vi "Cleaned RTK Multiple String Capture Software.vi"() -> ()   [LabVIEW 2011]
uses:
  COM Port Control.ctl
  binary clusters control.ctl
  <vilib>/Utility/sysdir.llb/System Directory Type.ctl
panel:
  out "shutdown blocker":bool
  in  "Tab Control":T1(tab)
  in  "Update setup":bool
  in  "shutdown":bool
  in  "Base File Path":path caption="Base File Path (Destination that all RCVR files will be saved in)"
  in  "Time between samples (seconds)":u32=5 min=1 max=600 step=1
  in  "Number of hours to collect before starting new file":u16=1 min=1 max=24 step=1
  in  "Grennich Offset":dbl=-8.0 caption="Greenwich offset (hours)" min=-12.0 max=12.0 step=1.0
  in  "UPDT COM 1":bool
  in  "Use RCVR 1":bool caption="Use RCVR"
  in  "Name of RCVR 1":string="RCVR 1" caption="Name of RCVR"
  in  "COM Port 1":T2={"flow control"=0, "COM Port"="", "parity"=enum."None", "data bits"=8, "baud rate"=9600} {"data bits" min=5 max=8 step=1; "flow control" items=["None", "XON/XOFF", "RTS/CTS", "XON/XOFF & RTS/CTS", "DTR/DSR", "XON/XOFF & DTR/DSR"]}
  out "Last 10 RCVR 1":string[](array[string])
  in  "A_Off R 1":dbl caption="Antenna offset (meters)" max=0.0 format="%.4g"
  in  "Name of RCVR 2":string="RCVR 2" caption="Name of RCVR"
  in  "UPDT COM 2":bool
  out "Last 10 RCVR 2":string[](array[string])
  in  "COM Port 2":T2={"flow control"=0, "COM Port"="", "parity"=enum."None", "data bits"=8, "baud rate"=9600} {"data bits" min=5 max=8 step=1; "flow control" items=["None", "XON/XOFF", "RTS/CTS", "XON/XOFF & RTS/CTS", "DTR/DSR", "XON/XOFF & DTR/DSR"]}
  in  "Use RCVR 2":bool caption="Use RCVR"
  in  "A_Off R 2":dbl caption="Antenna offset (meters)" max=0.0 format="%.4g"
  in  "Name of RCVR 3":string="RCVR 3" caption="Name of RCVR"
  in  "UPDT COM 3":bool
  out "Last 10 RCVR 3":string[](array[string])
  in  "COM Port 3":T2={"flow control"=0, "COM Port"="", "parity"=enum."None", "data bits"=8, "baud rate"=9600} {"data bits" min=5 max=8 step=1; "flow control" items=["None", "XON/XOFF", "RTS/CTS", "XON/XOFF & RTS/CTS", "DTR/DSR", "XON/XOFF & DTR/DSR"]}
  in  "Use RCVR 3":bool caption="Use RCVR"
  in  "A_Off R 3":dbl caption="Antenna offset (meters)" max=0.0 format="%.4g"
  in  "Name of RCVR 4":string="RCVR 4" caption="Name of RCVR"
  in  "UPDT COM 4":bool
  out "Last 10 RCVR 4":string[](array[string])
  in  "COM Port 4":T2={"flow control"=0, "COM Port"="", "parity"=enum."None", "data bits"=8, "baud rate"=9600} {"data bits" min=5 max=8 step=1; "flow control" items=["None", "XON/XOFF", "RTS/CTS", "XON/XOFF & RTS/CTS", "DTR/DSR", "XON/XOFF & DTR/DSR"]}
  in  "Use RCVR 4":bool caption="Use RCVR"
  in  "A_Off R 4":dbl caption="Antenna offset (meters)" max=0.0 format="%.4g"
  in  "Name of RCVR 5":string="RCVR 5" caption="Name of RCVR"
  in  "UPDT COM 5":bool
  out "Last 10 RCVR 5":string[](array[string])
  in  "COM Port 5":T2={"flow control"=0, "COM Port"="", "parity"=enum."None", "data bits"=8, "baud rate"=9600} {"data bits" min=5 max=8 step=1; "flow control" items=["None", "XON/XOFF", "RTS/CTS", "XON/XOFF & RTS/CTS", "DTR/DSR", "XON/XOFF & DTR/DSR"]}
  in  "A_Off R 5":dbl caption="Antenna offset (meters)" max=0.0 format="%.4g"
  in  "Use RCVR 5":bool caption="Use RCVR"
  in  "Name of RCVR 6":string="RCVR 6" caption="Name of RCVR"
  in  "UPDT COM 6":bool
  out "Last 10 RCVR 6":string[](array[string])
  in  "COM Port 6":T2={"flow control"=0, "COM Port"="", "parity"=enum."None", "data bits"=8, "baud rate"=9600} {"data bits" min=5 max=8 step=1; "flow control" items=["None", "XON/XOFF", "RTS/CTS", "XON/XOFF & RTS/CTS", "DTR/DSR", "XON/XOFF & DTR/DSR"]}
  in  "A_Off R 6":dbl caption="Antenna offset (meters)" max=0.0 format="%.4g"
  in  "Use RCVR 6":bool caption="Use RCVR"
  in  "Name of RCVR 7":string="RCVR 7" caption="Name of RCVR"
  in  "UPDT COM 7":bool
  out "Last 10 RCVR 7":string[](array[string])
  in  "COM Port 7":T2={"flow control"=0, "COM Port"="", "parity"=enum."None", "data bits"=8, "baud rate"=9600} {"data bits" min=5 max=8 step=1; "flow control" items=["None", "XON/XOFF", "RTS/CTS", "XON/XOFF & RTS/CTS", "DTR/DSR", "XON/XOFF & DTR/DSR"]}
  in  "A_Off R 7":dbl caption="Antenna offset (meters)" max=0.0 format="%.4g"
  in  "Use RCVR 7":bool caption="Use RCVR"
  in  "Name of RCVR 8":string="RCVR 8" caption="Name of RCVR"
  in  "UPDT COM 8":bool
  out "Last 10 RCVR 8":string[](array[string])
  in  "COM Port 8":T2={"flow control"=0, "COM Port"="", "parity"=enum."None", "data bits"=8, "baud rate"=9600} {"data bits" min=5 max=8 step=1; "flow control" items=["None", "XON/XOFF", "RTS/CTS", "XON/XOFF & RTS/CTS", "DTR/DSR", "XON/XOFF & DTR/DSR"]}
  in  "A_Off R 8":dbl caption="Antenna offset (meters)" max=0.0 format="%.4g"
  in  "Use RCVR 8":bool caption="Use RCVR"
  in  "Name of RCVR 9":string="RCVR 9" caption="Name of RCVR"
  in  "UPDT COM 9":bool
  out "Last 10 RCVR 9":string[](array[string])
  in  "COM Port 9":T2={"flow control"=0, "COM Port"="", "parity"=enum."None", "data bits"=8, "baud rate"=9600} {"data bits" min=5 max=8 step=1; "flow control" items=["None", "XON/XOFF", "RTS/CTS", "XON/XOFF & RTS/CTS", "DTR/DSR", "XON/XOFF & DTR/DSR"]}
  in  "A_Off R 9":dbl caption="Antenna offset (meters)" max=0.0 format="%.4g"
  in  "Use RCVR 9":bool caption="Use RCVR"
  in  "Name of RCVR 10":string="RCVR 10" caption="Name of RCVR"
  in  "UPDT COM 10":bool
  out "Last 10 RCVR 10":string[](array[string])
  in  "COM Port 10":T2={"flow control"=0, "COM Port"="", "parity"=enum."None", "data bits"=8, "baud rate"=9600} {"data bits" min=5 max=8 step=1; "flow control" items=["None", "XON/XOFF", "RTS/CTS", "XON/XOFF & RTS/CTS", "DTR/DSR", "XON/XOFF & DTR/DSR"]}
  in  "A_Off R 10":dbl caption="Antenna offset (meters)" max=0.0 format="%.4g"
  in  "Use RCVR 10":bool caption="Use RCVR"
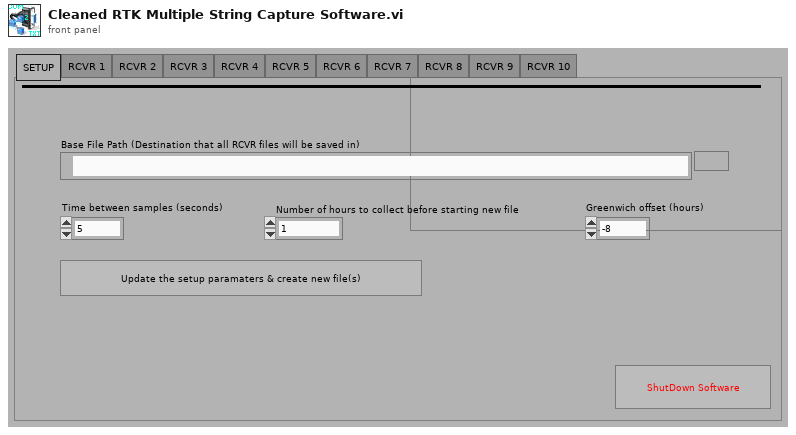
[diagram p1: front panel]
types:
  T1 = enum32{"SETUP", "RCVR 1", "RCVR 2", "RCVR 3", "RCVR 4", "RCVR 5", "RCVR 6", "RCVR 7", "RCVR 8", "RCVR 9", "RCVR 10"}
  T2 = typedef "COM Port Control.ctl" = cluster{"flow control":u16, "COM Port":refnum<visa-resource-name>, "parity":enum16{"None", "Odd", "Even", "Mark", "Space"}, "data bits":u16, "baud rate":u32}
  T3 = typedef "binary clusters control.ctl" = cluster{"setup save cluster":cluster{"Base File Path":path, "Time between samples (seconds)":u32, "Number of hours To Collect before starting new file ":u16, "Grennich Offset":dbl}, "RCVR1 Save Cluster":cluster{"Use RCVR 1":bool, "COM Port 1":T2, "Name of RCVR 1":string, "Antenna offset RCVR 1":dbl}, "RCVR2 Save cluster":cluster{"Use RCVR 2":bool, "COM Port 2":T2, "Name of RCVR 2":string, "Antenna offset RCVR 2":dbl}, "RCVR3 Save Cluster":cluster{"Use RCVR 3":bool, "Name of RCVR 3":string, "COM Port 3":T2, "Antenna offset RCVR 3":dbl}, "RCVR4 Save Cluster":cluster{"Use RCVR 4":bool, "Name of RCVR 4":string, "COM Port 4":T2, "Antenna offset RCVR 4":dbl}, "RCVR5 Save Cluster":cluster{"Use RCVR 5":bool, "Name of RCVR 5":string, "COM Port 5":T2, "Antenna offset RCVR 5":dbl}, "RCVR6 Save Cluster":cluster{"Use RCVR 6":bool, "Name of RCVR 6":string, "COM Port 6":T2, "Antenna offset RCVR 6":dbl}, "RCVR7 Save Cluster":cluster{"Use RCVR 7":bool, "Name of RCVR 7":string, "COM Port 7":T2, "Antenna offset RCVR 7":dbl}, "RCVR8 Save Cluster":cluster{"Use RCVR 8":bool, "Name of RCVR 8":string, "COM Port 8":T2, "Antenna offset RCVR 8":dbl}, "RCVR9 Save Cluster":cluster{"Use RCVR 9":bool, "Name of RCVR 9":string, "COM Port 9":T2, "Antenna offset RCVR 9":dbl}, "RCVR10 Save Cluster":cluster{"Use RCVR 10":bool, "Name of RCVR 10":string, "COM Port 10":T2, "Antenna offset RCVR 10":dbl}}
  T4 = enum16{"big-endian, network order", "native, host order", "little-endian"}
  T5 = cluster{"Number of hours To Collect before starting new file ":u16, "Base File Path":path, "Update setup":bool, "Shutdown software":bool, "Time between samples (seconds)":u32}
  T6 = typedef "System Directory Type.ctl" = i32
  T7 = cluster{"Base File Path":path, "Time between samples (seconds)":u32, "Number of hours To Collect before starting new file ":u16, "Grennich Offset":dbl}
  T8 = cluster{"Use RCVR 10":bool, "Name of RCVR 10":string, "COM Port 10":T2, "Antenna offset RCVR 10":dbl}
  T9 = cluster{"Use RCVR 1":bool, "COM Port 1":T2, "Name of RCVR 1":string, "Antenna offset RCVR 1":dbl}
  T10 = cluster{"Use RCVR 3":bool, "Name of RCVR 3":string, "COM Port 3":T2, "Antenna offset RCVR 3":dbl}
  T11 = cluster{"Use RCVR 4":bool, "Name of RCVR 4":string, "COM Port 4":T2, "Antenna offset RCVR 4":dbl}
  T12 = cluster{"Use RCVR 5":bool, "Name of RCVR 5":string, "COM Port 5":T2, "Antenna offset RCVR 5":dbl}
  T13 = cluster{"Use RCVR 6":bool, "Name of RCVR 6":string, "COM Port 6":T2, "Antenna offset RCVR 6":dbl}
  T14 = cluster{"Use RCVR 7":bool, "Name of RCVR 7":string, "COM Port 7":T2, "Antenna offset RCVR 7":dbl}
  T15 = cluster{"Use RCVR 8":bool, "Name of RCVR 8":string, "COM Port 8":T2, "Antenna offset RCVR 8":dbl}
  T16 = cluster{"Use RCVR 9":bool, "Name of RCVR 9":string, "COM Port 9":T2, "Antenna offset RCVR 9":dbl}
  T17 = cluster{"Use RCVR 2":bool, "COM Port 2":T2, "Name of RCVR 2":string, "Antenna offset RCVR 2":dbl}
  T18 = enum32{"invalid app kind", "Development System", "Run Time System", "Student Edition", "Embedded LabVIEW", "Evaluation", "Custom"}
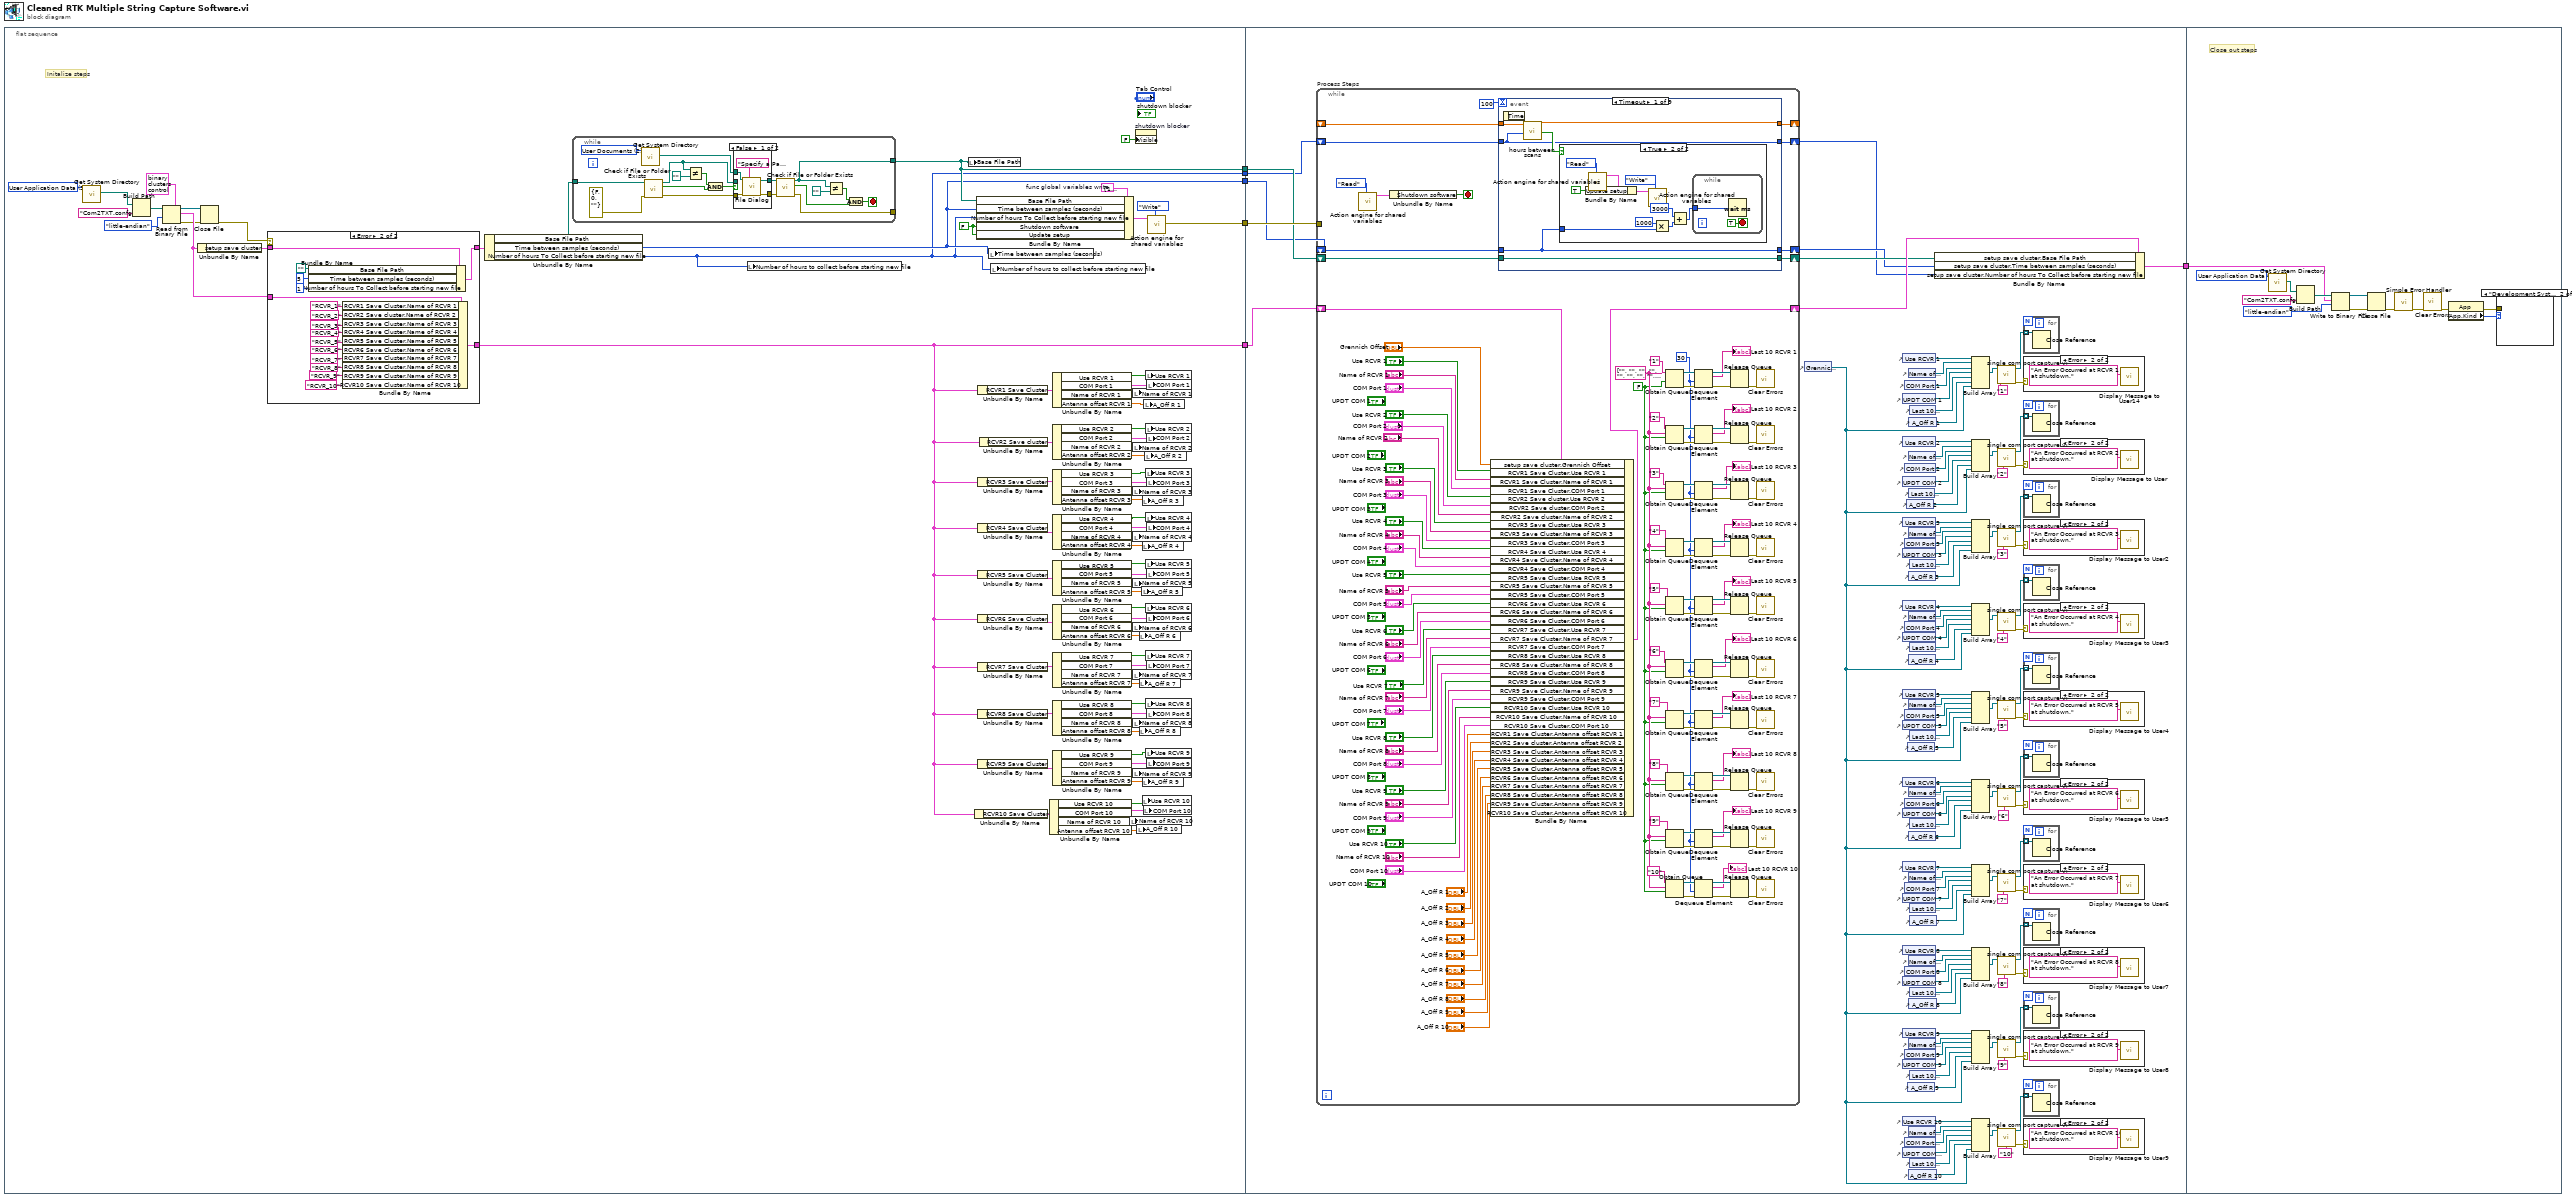
[diagram p0: block diagram]
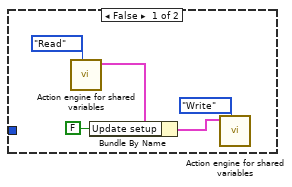
[diagram p14: hidden frame]
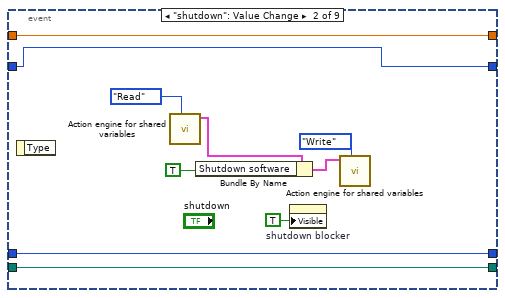
[diagram p15: hidden frame]
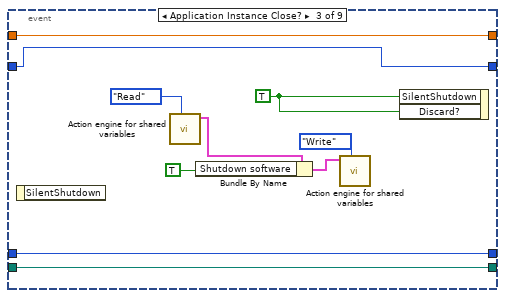
[diagram p16: hidden frame]
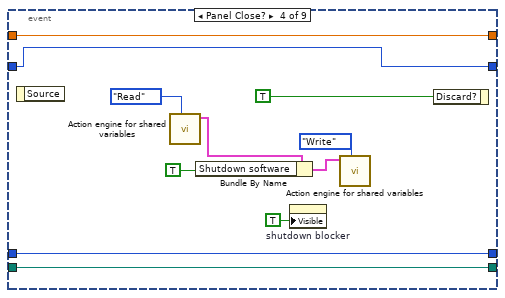
[diagram p17: hidden frame]
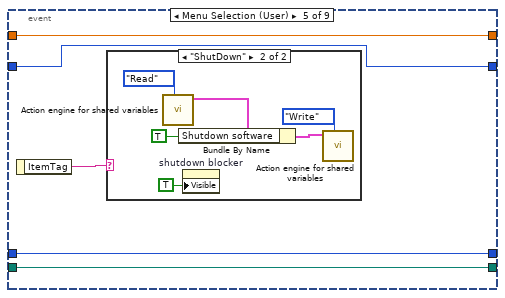
[diagram p18: hidden frame]
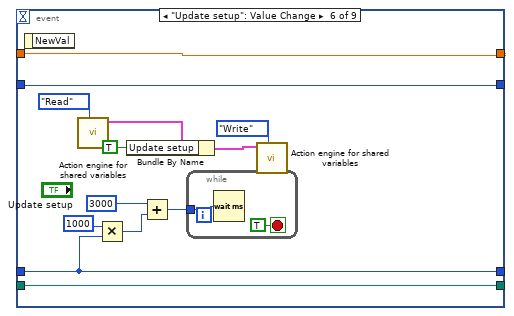
[diagram p20: hidden frame]
diagram:
  n1 = flat-sequence {
    tunnel: [w21] -> w5
    tunnel: [w20] -> w4
    tunnel: [w19] -> w3
    tunnel: [w18] -> w2
    tunnel: [w17] -> w1
    tunnel: [w216] -> w6
    tunnel: w5 -> [w221]
    tunnel: w4 -> [w167]
    tunnel: w3 -> [w166]
    tunnel: w2 -> [w165]
    tunnel: w1 -> [w164]
    tunnel: w6 -> [w487]
    frame #0 {
      w39 = FALSE ("Shutdown software")
      w37 = T5 {"Number of hours To Collect before starting new file "=1, "Base File Path"=path "", "Update setup"=TRUE, "Shutdown software"=TRUE, "Time between samples (seconds)"=5}  # func global variables write
      w22 = T6 3 items=["User Home"=0, "User Desktop"=1, "User Documents"=2, "User Application Data"=3, "User Preferences"=4, "User Temporary"=5, "Public Documents"=6, "Public Application Data"=7, "Public Preferences"=8, "Public Cache"=13, "System Core Libraries"=9, "System Installed Libraries"=10, "Application Files"=11, "Boot Volume Root"=12] ("system directory type")
      # "Initalize steps"
      n2 = call <vilib>:"Get System Directory.vi"("system directory type"=w22) -> ("system directory"=w23:path)  [unwired: 10 in]
      n3 = Build Path(base path=w23, name or relative path="Com2TXT.confg") -> (appended path=w29:path)
      n4 = Read from Binary File(5:T3 {"setup save cluster"={"Base File Path"=path "", "Time between samples (seconds)"=0, "Number of hours To Collect before starting new file "=0, "Grennich Offset"=0.0}, "RCVR1 Save Cluster"={"Use RCVR 1"=FALSE, "COM Port 1"={"flow control"=0, "COM Port"="", "parity"=enum."None", "data bits"=0, "baud rate"=0}, "Name of RCVR 1"="", "Antenna offset RCVR 1"=0.0}, "RCVR2 Save cluster"={"Use RCVR 2"=FALSE, "COM Port 2"={"flow control"=0, "COM Port"="", "parity"=enum."None", "data bits"=0, "baud rate"=0}, "Name of RCVR 2"="", "Antenna offset RCVR 2"=0.0}, "RCVR3 Save Cluster"={"Use RCVR 3"=FALSE, "Name of RCVR 3"="", "COM Port 3"={"flow control"=0, "COM Port"="", "parity"=enum."None", "data bits"=0, "baud rate"=0}, "Antenna offset RCVR 3"=0.0}, "RCVR4 Save Cluster"={"Use RCVR 4"=FALSE, "Name of RCVR 4"="", "COM Port 4"={"flow control"=0, "COM Port"="", "parity"=enum."None", "data bits"=0, "baud rate"=0}, "Antenna offset RCVR 4"=0.0}, "RCVR5 Save Cluster"={"Use RCVR 5"=FALSE, "Name of RCVR 5"="", "COM Port 5"={"flow control"=0, "COM Port"="", "parity"=enum."None", "data bits"=0, "baud rate"=0}, "Antenna offset RCVR 5"=0.0}, "RCVR6 Save Cluster"={"Use RCVR 6"=FALSE, "Name of RCVR 6"="", "COM Port 6"={"flow control"=0, "COM Port"="", "parity"=enum."None", "data bits"=0, "baud rate"=0}, "Antenna offset RCVR 6"=0.0}, "RCVR7 Save Cluster"={"Use RCVR 7"=FALSE, "Name of RCVR 7"="", "COM Port 7"={"flow control"=0, "COM Port"="", "parity"=enum."None", "data bits"=0, "baud rate"=0}, "Antenna offset RCVR 7"=0.0}, "RCVR8 Save Cluster"={"Use RCVR 8"=FALSE, "Name of RCVR 8"="", "COM Port 8"={"flow control"=0, "COM Port"="", "parity"=enum."None", "data bits"=0, "baud rate"=0}, "Antenna offset RCVR 8"=0.0}, "RCVR9 Save Cluster"={"Use RCVR 9"=FALSE, "Name of RCVR 9"="", "COM Port 9"={"flow control"=0, "COM Port"="", "parity"=enum."None", "data bits"=0, "baud rate"=0}, "Antenna offset RCVR 9"=0.0}, "RCVR10 Save Cluster"={"Use RCVR 10"=FALSE, "Name of RCVR 10"="", "COM Port 10"={"flow control"=0, "COM Port"="", "parity"=enum."None", "data bits"=0, "baud rate"=0}, "Antenna offset RCVR 10"=0.0}} ("output cluster"), 9:T4."little-endian" ("byte order (0:big-endian, network order)"), 11:w29) -> (0:w26:errorcluster, 2:w34:T3, 3:w27:refnum<file>)  [unwired: 3 in, 1 out]
      n5 = Unbundle By Name(w34) -> ("setup save cluster"=w31:T7)
      n6 = Close File(refnum=w27, error in=w26) -> (error out=w33:errorcluster)  [unwired: 1 out]
      n7 = case shown="Error" w33 {
        tunnel: w31 -> [w81 w98]
        tunnel: [w81 w97] -> w32
        tunnel: [w80 w94] -> w21
        tunnel: w34 -> [w80 w93]
        frame No Error {
        }
        frame Error {
          n8 = Bundle By Name(cluster=w98, "Base File Path"=path "", "Time between samples (seconds)"=u32 5, "Number of hours To Collect before starting new file"=u16 1) -> (w97:T7)
          n9 = Bundle By Name(cluster=w93, "RCVR1 Save Cluster.Name of RCVR 1"="RCVR_1", "RCVR2 Save cluster.Name of RCVR 2"="RCVR_2" ("RCVR1 Save Cluster.Name of RCVR 1"), "RCVR3 Save Cluster.Name of RCVR 3"="RCVR_3" ("RCVR1 Save Cluster.Name of RCVR 1"), "RCVR4 Save Cluster.Name of RCVR 4"="RCVR_4" ("RCVR1 Save Cluster.Name of RCVR 1"), "RCVR5 Save Cluster.Name of RCVR 5"="RCVR_5" ("RCVR1 Save Cluster.Name of RCVR 1"), "RCVR6 Save Cluster.Name of RCVR 6"="RCVR_6" ("RCVR1 Save Cluster.Name of RCVR 1"), "RCVR7 Save Cluster.Name of RCVR 7"="RCVR_7" ("RCVR1 Save Cluster.Name of RCVR 1"), "RCVR8 Save Cluster.Name of RCVR 8"="RCVR_8" ("RCVR1 Save Cluster.Name of RCVR 1"), "RCVR9 Save Cluster.Name of RCVR 9"="RCVR_9" ("RCVR1 Save Cluster.Name of RCVR 1"), "RCVR10 Save Cluster.Name of RCVR 10"="RCVR_10" ("RCVR1 Save Cluster.Name of RCVR 1")) -> (w94:T3)
        }
      }
      n10 = Unbundle By Name(w32) -> ("Base File Path"=w25:path, "Time between samples (seconds)"=w18:u32, "Number of hours To Collect before starting new file"=w17:u16)
      n11 = while {
        tunnel: [w110] -> w19
        tunnel: [w112] -> _
        tunnel: w25 -> [w101]
        stop <- w111 stop-if-true
        w100 = T6 2 items=["User Home"=0, "User Desktop"=1, "User Documents"=2, "User Application Data"=3, "User Preferences"=4, "User Temporary"=5, "Public Documents"=6, "Public Application Data"=7, "Public Preferences"=8, "Public Cache"=13, "System Core Libraries"=9, "System Installed Libraries"=10, "Application Files"=11, "Boot Volume Root"=12] ("system directory type")
        n12 = call <vilib>:"Get System Directory.vi"("system directory type"=w100) -> ("system directory"=w99:path)  [unwired: 10 in]
        n13 = call <vilib>:"Check if File or Folder Exists.vi"("error in (no error)"=errorcluster {"status"=FALSE, "code"=0, "source"=""}, "path"=w101) -> ("error out"=w114:errorcluster, "file or folder exists?"=w104:bool, "dup path"=w103:path)  [unwired: 7 in]
        n14 = Not Equal?(x=w103, y=path "") -> (x != y?=w106:bool)
        n15 = And(x=w106, y=w104) -> (x .and. y?=w102:bool)
        n16 = case shown="False" w102 {
          tunnel: [w121 w123] -> w116
          tunnel: w103 -> [_ w123]
          tunnel: w114 -> [w120 w122]
          tunnel: [w119 w122] -> w113
          tunnel: w99 -> [w117 _]
          frame False {
            n17 = call "File Dialog"("start path"=w117, "prompt"="Specify a Path to Save RCVR .TXT files", "error in"=w120) -> ("selected path"=w121:path, "error out"=w119:errorcluster)  [unwired: 9 in, 2 out]
          }
          frame True {
          }
        }
        n18 = call <vilib>:"Check if File or Folder Exists.vi"("error in (no error)"=w113, "path"=w116) -> ("error out"=w112:errorcluster, "file or folder exists?"=w107:bool, "dup path"=w110:path)  [unwired: 7 in]
        n19 = Not Equal?(x=w110, y=path "") -> (x != y?=w108:bool)
        n20 = And(x=w108, y=w107) -> (x .and. y?=w111:bool)
      }
      n21 = local write "Number of hours to collect before starting new file"(w17) -> ()
      n22 = local write "Base File Path"(w19) -> ()
      n23 = Unbundle By Name(w21) -> ("RCVR10 Save Cluster"=w78:T8)
      n24 = Bundle By Name(cluster=w37, "Base File Path"=w19, "Time between samples (seconds)"=w18, "Number of hours To Collect before starting new file"=w17, "Shutdown software"=w39, "Update setup"=w39) -> (w36:T5)
      n25 = Unbundle By Name(w21) -> ("RCVR1 Save Cluster"=w79:T9)
      n26 = Unbundle By Name(w21) -> ("RCVR3 Save Cluster"=w71:T10)
      n27 = Unbundle By Name(w21) -> ("RCVR4 Save Cluster"=w72:T11)
      n28 = Unbundle By Name(w21) -> ("RCVR5 Save Cluster"=w73:T12)
      n29 = Unbundle By Name(w21) -> ("RCVR6 Save Cluster"=w74:T13)
      n30 = Unbundle By Name(w21) -> ("RCVR7 Save Cluster"=w75:T14)
      n31 = Unbundle By Name(w21) -> ("RCVR8 Save Cluster"=w76:T15)
      n32 = Unbundle By Name(w21) -> ("RCVR9 Save Cluster"=w77:T16)
      n33 = Unbundle By Name(w21) -> ("RCVR2 Save cluster"=w70:T17)
      n34 = local write "Time between samples (seconds)"(w18) -> ()
      n35 = local write "Number of hours to collect before starting new file"(w17) -> ()
      n36 = Unbundle By Name(w78) -> ("Use RCVR 10"=w63:bool, "COM Port 10"=w62:T2, "Name of RCVR 10"=w61:string, "Antenna offset RCVR 10"=w7:dbl)
      n37 = Unbundle By Name(w79) -> ("Use RCVR 1"=w64:bool, "COM Port 1"=w65:T2, "Name of RCVR 1"=w66:string, "Antenna offset RCVR 1"=w16:dbl)
      n38 = Unbundle By Name(w70) -> ("Use RCVR 2"=w67:bool, "COM Port 2"=w68:T2, "Name of RCVR 2"=w69:string, "Antenna offset RCVR 2"=w15:dbl)
      n39 = Unbundle By Name(w71) -> ("Use RCVR 3"=w40:bool, "COM Port 3"=w41:T2, "Name of RCVR 3"=w42:string, "Antenna offset RCVR 3"=w14:dbl)
      n40 = Unbundle By Name(w72) -> ("Use RCVR 4"=w45:bool, "COM Port 4"=w44:T2, "Name of RCVR 4"=w43:string, "Antenna offset RCVR 4"=w13:dbl)
      n41 = Unbundle By Name(w73) -> ("Use RCVR 5"=w46:bool, "COM Port 5"=w47:T2, "Name of RCVR 5"=w48:string, "Antenna offset RCVR 5"=w12:dbl)
      n42 = Unbundle By Name(w74) -> ("Use RCVR 6"=w51:bool, "COM Port 6"=w50:T2, "Name of RCVR 6"=w49:string, "Antenna offset RCVR 6"=w11:dbl)
      n43 = Unbundle By Name(w75) -> ("Use RCVR 7"=w52:bool, "COM Port 7"=w53:T2, "Name of RCVR 7"=w54:string, "Antenna offset RCVR 7"=w10:dbl)
      n44 = Unbundle By Name(w76) -> ("Use RCVR 8"=w57:bool, "COM Port 8"=w56:T2, "Name of RCVR 8"=w55:string, "Antenna offset RCVR 8"=w9:dbl)
      n45 = Unbundle By Name(w77) -> ("Use RCVR 9"=w58:bool, "COM Port 9"=w59:T2, "Name of RCVR 9"=w60:string, "Antenna offset RCVR 9"=w8:dbl)
      n46 = local write "Name of RCVR 10"(w61) -> ()
      n47 = local write "Name of RCVR 1"(w66) -> ()
      n48 = local write "Name of RCVR 2"(w69) -> ()
      n49 = local write "Name of RCVR 3"(w42) -> ()
      n50 = local write "Name of RCVR 4"(w43) -> ()
      n51 = local write "Name of RCVR 5"(w48) -> ()
      n52 = local write "Name of RCVR 6"(w49) -> ()
      n53 = local write "Name of RCVR 7"(w54) -> ()
      n54 = local write "Name of RCVR 8"(w55) -> ()
      n55 = local write "Name of RCVR 9"(w60) -> ()
      n56 = property on="shutdown blocker" class="Bool (strict)"("Visible"=FALSE) -> ()  [unwired: 2 in, 2 out]
      n57 = local write "A_Off R 10"(w7) -> ()
      n58 = local write "A_Off R 6"(w11) -> ()
      n59 = local write "A_Off R 7"(w10) -> ()
      n60 = local write "A_Off R 8"(w9) -> ()
      n61 = local write "A_Off R 5"(w12) -> ()
      n62 = local write "A_Off R 3"(w14) -> ()
      n63 = local write "A_Off R 4"(w13) -> ()
      n64 = local write "A_Off R 9"(w8) -> ()
      n65 = local write "Use RCVR 10"(w63) -> ()
      n66 = local write "COM Port 10"(w62) -> ()
      n67 = local write "A_Off R 1"(w16) -> ()
      n68 = local write "A_Off R 2"(w15) -> ()
      n69 = local write "Use RCVR 1"(w64) -> ()
      n70 = local write "Use RCVR 2"(w67) -> ()
      n71 = local write "Use RCVR 3"(w40) -> ()
      n72 = local write "Use RCVR 4"(w45) -> ()
      n73 = local write "Use RCVR 5"(w46) -> ()
      n74 = local write "Use RCVR 6"(w51) -> ()
      n75 = local write "Use RCVR 7"(w52) -> ()
      n76 = local write "Use RCVR 8"(w57) -> ()
      n77 = local write "Use RCVR 9"(w58) -> ()
      n78 = local write "COM Port 1"(w65) -> ()
      n79 = local write "COM Port 2"(w68) -> ()
      n80 = local write "COM Port 3"(w41) -> ()
      n81 = local write "COM Port 4"(w44) -> ()
      n82 = local write "COM Port 5"(w47) -> ()
      n83 = local write "COM Port 6"(w50) -> ()
      n84 = local write "COM Port 7"(w53) -> ()
      n85 = local write "COM Port 8"(w56) -> ()
      n86 = local write "COM Port 9"(w59) -> ()
      n87 = call "Action engine for shared variables.vi"("read/write"=enum16{"Read", "Write"}."Write", "func global variables write"=w36) -> ("error out"=w20:errorcluster)  [unwired: 8 in, 1 out]
    }
    frame #1 {
      n88 = while "Process Steps" {
        shift-right: [w381] -> _
        shift-left: _ -> [w380]
        shift-right: [w344] -> w217
        shift-left: w164 -> [w343]
        shift-right: [w342] -> w218
        shift-left: w165 -> [w341]
        shift-right: [w345] -> w220
        shift-left: w221 -> [w373]
        shift-right: [w340] -> w219
        shift-left: w166 -> [w339]
        tunnel: w167 -> [_]
        stop <- w377 stop-if-true
        w268 = 30 ("timeout in ms (-1)")
        w266 = FALSE ("create if not found? (T)")
        w267 = string[] ["", "", "", "", "", "", "", "", "", ""] ("Last 10 RCVR 1")
        n89 = call "Action engine for shared variables.vi"("read/write"=enum16{"Read", "Write"}."Read") -> ("func global variables read"=w378:T5)  [unwired: 9 in, 1 out]
        n90 = Unbundle By Name(w378) -> ("Shutdown software"=w377:bool)
        n91 = Bundle By Name(cluster=w373, "setup save cluster.Grennich Offset"="Grennich Offset", "RCVR1 Save Cluster.Use RCVR 1"="Use RCVR 1", "RCVR1 Save Cluster.Name of RCVR 1"="Name of RCVR 1", "RCVR1 Save Cluster.COM Port 1"="COM Port 1", "RCVR2 Save cluster.Use RCVR 2"="Use RCVR 2", "RCVR2 Save cluster.COM Port 2"="COM Port 2", "RCVR2 Save cluster.Name of RCVR 2"="Name of RCVR 2", "RCVR3 Save Cluster.Use RCVR 3"="Use RCVR 3", "RCVR3 Save Cluster.Name of RCVR 3"="Name of RCVR 3", "RCVR3 Save Cluster.COM Port 3"="COM Port 3", "RCVR4 Save Cluster.Use RCVR 4"="Use RCVR 4", "RCVR4 Save Cluster.Name of RCVR 4"="Name of RCVR 4", "RCVR4 Save Cluster.COM Port 4"="COM Port 4", "RCVR5 Save Cluster.Use RCVR 5"="Use RCVR 5", "RCVR5 Save Cluster.Name of RCVR 5"="Name of RCVR 5", "RCVR5 Save Cluster.COM Port 5"="COM Port 5", "RCVR6 Save Cluster.Use RCVR 6"="Use RCVR 6", "RCVR6 Save Cluster.Name of RCVR 6"="Name of RCVR 6", "RCVR6 Save Cluster.COM Port 6"="COM Port 6", "RCVR7 Save Cluster.Use RCVR 7"="Use RCVR 7", "RCVR7 Save Cluster.Name of RCVR 7"="Name of RCVR 7", "RCVR7 Save Cluster.COM Port 7"="COM Port 7", "RCVR8 Save Cluster.Use RCVR 8"="Use RCVR 8", "RCVR8 Save Cluster.Name of RCVR 8"="Name of RCVR 8", "RCVR8 Save Cluster.COM Port 8"="COM Port 8", "RCVR9 Save Cluster.Use RCVR 9"="Use RCVR 9", "RCVR9 Save Cluster.Name of RCVR 9"="Name of RCVR 9", "RCVR9 Save Cluster.COM Port 9"="COM Port 9", "RCVR10 Save Cluster.Use RCVR 10"="Use RCVR 10", "RCVR10 Save Cluster.Name of RCVR 10"="Name of RCVR 10", "RCVR10 Save Cluster.COM Port 10"="COM Port 10", "RCVR1 Save Cluster.Antenna offset RCVR 1"="A_Off R 1", "RCVR2 Save cluster.Antenna offset RCVR 2"="A_Off R 2", "RCVR3 Save Cluster.Antenna offset RCVR 3"="A_Off R 3", "RCVR4 Save Cluster.Antenna offset RCVR 4"="A_Off R 4", "RCVR5 Save Cluster.Antenna offset RCVR 5"="A_Off R 5", "RCVR6 Save Cluster.Antenna offset RCVR 6"="A_Off R 6", "RCVR7 Save Cluster.Antenna offset RCVR 7"="A_Off R 7", "RCVR8 Save Cluster.Antenna offset RCVR 8"="A_Off R 8", "RCVR9 Save Cluster.Antenna offset RCVR 9"="A_Off R 9", "RCVR10 Save Cluster.Antenna offset RCVR 10"="A_Off R 10") -> (w345:T3)
        n92 = event shown="[0] Timeout" {
          selector: _ -> [_ _ _ _ _ _ _ _ _]
          dyn-events: _ -> [_ _ _ _ _ _ _ _ _]
          timeout: 100 -> [_ _ _ _ _ _ _ _ _]
          tunnel: [w387 w414 w425 w435 w440 w456 w470 w478 w486] -> w381
          tunnel: w380 -> [w386 w414 w425 w435 w440 w456 w470 w478 w486]
          tunnel: [w385 w410 w421 w431 w439 w452 w467 w475 "Number of hours to collect before starting new file"] -> w344
          tunnel: w343 -> [w385 w410 w421 w431 w439 w452 w467 w475 _]
          tunnel: [w384 w409 w420 w430 w438 w450 w466 "Time between samples (seconds)" w482] -> w342
          tunnel: w341 -> [w384 w409 w420 w430 w438 w450 w466 _ w482]
          tunnel: [w383 w408 w419 w429 w437 w451 "Base File Path" w473 w481] -> w340
          tunnel: w339 -> [w383 w408 w419 w429 w437 w451 _ w473 w481]
          event Timeout {
            n93 = event-data() -> ()  [unwired: 1 in, 1 out]
            n94 = call "hours between scans.vi"("Number of hours To Collect before starting new file"=w385, "Input start time"=w386) -> ("Time has Elapsed"=w388:bool, "output next start time"=w387:dbl)  [unwired: 7 in, 1 out]
            n95 = case shown="True" w388 {
              tunnel: w384 -> [_ w403]
              frame False {
                n96 = call "Action engine for shared variables.vi"("read/write"=enum16{"Read", "Write"}."Read") -> ("func global variables read"=w389:T5)  [unwired: 9 in, 1 out]
                n97 = Bundle By Name(cluster=w389, "Update setup"=FALSE) -> (w391:T5)
                n98 = call "Action engine for shared variables.vi"("read/write"=enum16{"Read", "Write"}."Write", "func global variables write"=w391) -> ()  [unwired: 8 in, 2 out]
              }
              frame True {
                n99 = call "Action engine for shared variables.vi"("read/write"=enum16{"Read", "Write"}."Read") -> ("func global variables read"=w394:T5)  [unwired: 9 in, 1 out]
                n100 = Bundle By Name(cluster=w394, "Update setup"=TRUE) -> (w396:T5)
                n101 = call "Action engine for shared variables.vi"("read/write"=enum16{"Read", "Write"}."Write", "func global variables write"=w396) -> ()  [unwired: 8 in, 2 out]
                n102 = Multiply(x=u32 1000, y=w403) -> (x*y=w401:u32)
                n103 = Add(x=u32 3000 ("milliseconds to wait"), y=w401) -> (x+y=w399:u32)
                n104 = while {
                  tunnel: w399 -> [w404]
                  stop <- TRUE ("stop 2") stop-if-true
                  n105 = Wait (ms)(milliseconds to wait=w404) -> ()  [unwired: 1 out]
                }
              }
            }
          }
          event "shutdown": Value Change {
            n106 = event-data() -> ()  [unwired: 1 in, 1 out]
            n107 = call "Action engine for shared variables.vi"("read/write"=enum16{"Read", "Write"}."Read") -> ("func global variables read"=w407:T5)  [unwired: 9 in, 1 out]
            n108 = Bundle By Name(cluster=w407, "Shutdown software"=TRUE ("Update setup")) -> (w411:T5)
            n109 = property on="shutdown blocker" class="Bool (strict)"("Visible"=TRUE) -> ()  [unwired: 2 in, 2 out]
            n110 = call "Action engine for shared variables.vi"("read/write"=enum16{"Read", "Write"}."Write", "func global variables write"=w411) -> ()  [unwired: 8 in, 2 out]
          }
          event Application Instance Close? {
            w416 = TRUE ("SilentShutdown")
            n111 = event-data() -> ()  [unwired: 1 in, 1 out]
            n112 = call "Action engine for shared variables.vi"("read/write"=enum16{"Read", "Write"}."Read") -> ("func global variables read"=w418:T5)  [unwired: 9 in, 1 out]
            n113 = Bundle By Name(cluster=w418, "Shutdown software"=TRUE ("Update setup")) -> (w422:T5)
            n114 = call "Action engine for shared variables.vi"("read/write"=enum16{"Read", "Write"}."Write", "func global variables write"=w422) -> ()  [unwired: 8 in, 2 out]
            n115 = event-data("SilentShutdown"=w416, "Discard?"=w416) -> ()  [unwired: 1 in, 1 out]
          }
          event Panel Close? {
            n116 = event-data() -> ()  [unwired: 1 in, 1 out]
            n117 = call "Action engine for shared variables.vi"("read/write"=enum16{"Read", "Write"}."Read") -> ("func global variables read"=w428:T5)  [unwired: 9 in, 1 out]
            n118 = Bundle By Name(cluster=w428, "Shutdown software"=TRUE ("Update setup")) -> (w432:T5)
            n119 = property on="shutdown blocker" class="Bool (strict)"("Visible"=TRUE) -> ()  [unwired: 2 in, 2 out]
            n120 = call "Action engine for shared variables.vi"("read/write"=enum16{"Read", "Write"}."Write", "func global variables write"=w432) -> ()  [unwired: 8 in, 2 out]
            n121 = event-data("Discard?"=TRUE ("SilentShutdown")) -> ()  [unwired: 1 in, 1 out]
          }
          event Menu Selection (User) {
            n122 = event-data() -> ("ItemTag"=w441:string)  [unwired: 1 in]
            n123 = case shown="\"ShutDown\"" w441 {
              frame "0", Default {
              }
              frame "ShutDown" {
                n124 = call "Action engine for shared variables.vi"("read/write"=enum16{"Read", "Write"}."Read") -> ("func global variables read"=w442:T5)  [unwired: 9 in, 1 out]
                n125 = Bundle By Name(cluster=w442, "Shutdown software"=TRUE ("Update setup")) -> (w444:T5)
                n126 = property on="shutdown blocker" class="Bool (strict)"("Visible"=TRUE) -> ()  [unwired: 2 in, 2 out]
                n127 = call "Action engine for shared variables.vi"("read/write"=enum16{"Read", "Write"}."Write", "func global variables write"=w444) -> ()  [unwired: 8 in, 2 out]
              }
            }
          }
          event "Update setup": Value Change {
            n128 = event-data() -> ()  [unwired: 1 in, 1 out]
            n129 = call "Action engine for shared variables.vi"("read/write"=enum16{"Read", "Write"}."Read") -> ("func global variables read"=w448:T5)  [unwired: 9 in, 1 out]
            n130 = Multiply(x=u32 1000, y=w450) -> (x*y=w460:u32)
            n131 = Bundle By Name(cluster=w448, "Update setup"=TRUE) -> (w453:T5)
            n132 = Add(x=u32 3000 ("milliseconds to wait"), y=w460) -> (x+y=w457:u32)
            n133 = while {
              tunnel: w457 -> [w461]
              stop <- TRUE ("stop 2") stop-if-true
              n134 = Wait (ms)(milliseconds to wait=w461) -> ()  [unwired: 1 out]
            }
            n135 = call "Action engine for shared variables.vi"("read/write"=enum16{"Read", "Write"}."Write", "func global variables write"=w453) -> ()  [unwired: 8 in, 2 out]
          }
          event "Base File Path": Value Change {
            n136 = event-data() -> ()  [unwired: 1 in, 1 out]
            n137 = call "Action engine for shared variables.vi"("read/write"=enum16{"Read", "Write"}."Read") -> ("func global variables read"=w463:T5)  [unwired: 9 in, 1 out]
            n138 = Bundle By Name(cluster=w463, "Base File Path"="Base File Path") -> (w468:T5)
            n139 = call "Action engine for shared variables.vi"("read/write"=enum16{"Read", "Write"}."Write", "func global variables write"=w468) -> ()  [unwired: 8 in, 2 out]
          }
          event "Time between samples (seconds)": Value Change {
            n140 = event-data() -> ()  [unwired: 1 in, 1 out]
            n141 = call "Action engine for shared variables.vi"("read/write"=enum16{"Read", "Write"}."Read") -> ("func global variables read"=w471:T5)  [unwired: 9 in, 1 out]
            n142 = Bundle By Name(cluster=w471, "Time between samples (seconds)"="Time between samples (seconds)") -> (w476:T5)
            n143 = call "Action engine for shared variables.vi"("read/write"=enum16{"Read", "Write"}."Write", "func global variables write"=w476) -> ()  [unwired: 8 in, 2 out]
          }
          event "Number of hours to collect before starting new file": Value Change {
            n144 = event-data() -> ()  [unwired: 1 in, 1 out]
            n145 = call "Action engine for shared variables.vi"("read/write"=enum16{"Read", "Write"}."Read") -> ("func global variables read"=w479:T5)  [unwired: 9 in, 1 out]
            n146 = Bundle By Name(cluster=w479, "Number of hours To Collect before starting new file"="Number of hours to collect before starting new file") -> (w484:T5)
            n147 = call "Action engine for shared variables.vi"("read/write"=enum16{"Read", "Write"}."Write", "func global variables write"=w484) -> ()  [unwired: 8 in, 2 out]
          }
        }
        n148 = Obtain Queue(name (unnamed)="1", element data type=w267, create if not found? (T)=w266) -> (queue out=w337:refnum<queue>, error out=w336:errorcluster)  [unwired: 2 in, 1 out]
        n149 = Obtain Queue(name (unnamed)="2", element data type=w267, create if not found? (T)=w266) -> (queue out=w327:refnum<queue>, error out=w328:errorcluster)  [unwired: 2 in, 1 out]
        n150 = Obtain Queue(name (unnamed)="3", element data type=w267, create if not found? (T)=w266) -> (queue out=w326:refnum<queue>, error out=w325:errorcluster)  [unwired: 2 in, 1 out]
        n151 = Obtain Queue(name (unnamed)="4", element data type=w267, create if not found? (T)=w266) -> (queue out=w317:refnum<queue>, error out=w318:errorcluster)  [unwired: 2 in, 1 out]
        n152 = Obtain Queue(name (unnamed)="5", element data type=w267, create if not found? (T)=w266) -> (queue out=w316:refnum<queue>, error out=w315:errorcluster)  [unwired: 2 in, 1 out]
        n153 = Obtain Queue(name (unnamed)="6", element data type=w267, create if not found? (T)=w266) -> (queue out=w307:refnum<queue>, error out=w308:errorcluster)  [unwired: 2 in, 1 out]
        n154 = Obtain Queue(name (unnamed)="7", element data type=w267, create if not found? (T)=w266) -> (queue out=w306:refnum<queue>, error out=w305:errorcluster)  [unwired: 2 in, 1 out]
        n155 = Obtain Queue(name (unnamed)="8", element data type=w267, create if not found? (T)=w266) -> (queue out=w297:refnum<queue>, error out=w298:errorcluster)  [unwired: 2 in, 1 out]
        n156 = Obtain Queue(name (unnamed)="9", element data type=w267, create if not found? (T)=w266) -> (queue out=w296:refnum<queue>, error out=w295:errorcluster)  [unwired: 2 in, 1 out]
        n157 = Obtain Queue(name (unnamed)="10", element data type=w267, create if not found? (T)=w266) -> (queue out=w287:refnum<queue>, error out=w288:errorcluster)  [unwired: 2 in, 1 out]
        n158 = Dequeue Element(queue=w337, timeout in ms (-1)=w268, error in (no error)=w336) -> (queue out=w335:refnum<queue>, element=→"Last 10 RCVR 1":string[], error out=w334:errorcluster)  [unwired: 1 out]
        n159 = Dequeue Element(queue=w327, timeout in ms (-1)=w268, error in (no error)=w328) -> (queue out=w329:refnum<queue>, element=→"Last 10 RCVR 2":string[], error out=w330:errorcluster)  [unwired: 1 out]
        n160 = Dequeue Element(queue=w326, timeout in ms (-1)=w268, error in (no error)=w325) -> (queue out=w324:refnum<queue>, element=→"Last 10 RCVR 3":string[], error out=w323:errorcluster)  [unwired: 1 out]
        n161 = Dequeue Element(queue=w317, timeout in ms (-1)=w268, error in (no error)=w318) -> (queue out=w319:refnum<queue>, element=→"Last 10 RCVR 4":string[], error out=w320:errorcluster)  [unwired: 1 out]
        n162 = Dequeue Element(queue=w316, timeout in ms (-1)=w268, error in (no error)=w315) -> (queue out=w314:refnum<queue>, element=→"Last 10 RCVR 5":string[], error out=w313:errorcluster)  [unwired: 1 out]
        n163 = Dequeue Element(queue=w307, timeout in ms (-1)=w268, error in (no error)=w308) -> (queue out=w309:refnum<queue>, element=→"Last 10 RCVR 6":string[], error out=w310:errorcluster)  [unwired: 1 out]
        n164 = Dequeue Element(queue=w306, timeout in ms (-1)=w268, error in (no error)=w305) -> (queue out=w304:refnum<queue>, element=→"Last 10 RCVR 7":string[], error out=w303:errorcluster)  [unwired: 1 out]
        n165 = Dequeue Element(queue=w297, timeout in ms (-1)=w268, error in (no error)=w298) -> (queue out=w299:refnum<queue>, element=→"Last 10 RCVR 8":string[], error out=w300:errorcluster)  [unwired: 1 out]
        n166 = Dequeue Element(queue=w296, timeout in ms (-1)=w268, error in (no error)=w295) -> (queue out=w294:refnum<queue>, element=→"Last 10 RCVR 9":string[], error out=w293:errorcluster)  [unwired: 1 out]
        n167 = Dequeue Element(queue=w287, timeout in ms (-1)=w268, error in (no error)=w288) -> (queue out=w289:refnum<queue>, element=→"Last 10 RCVR 10":string[], error out=w290:errorcluster)  [unwired: 1 out]
        n168 = Release Queue(queue=w335, error in (no error)=w334) -> (error out=w332:errorcluster)  [unwired: 1 in, 2 out]
        n169 = Release Queue(queue=w329, error in (no error)=w330) -> (error out=w331:errorcluster)  [unwired: 1 in, 2 out]
        n170 = Release Queue(queue=w324, error in (no error)=w323) -> (error out=w322:errorcluster)  [unwired: 1 in, 2 out]
        n171 = Release Queue(queue=w319, error in (no error)=w320) -> (error out=w321:errorcluster)  [unwired: 1 in, 2 out]
        n172 = Release Queue(queue=w314, error in (no error)=w313) -> (error out=w312:errorcluster)  [unwired: 1 in, 2 out]
        n173 = Release Queue(queue=w309, error in (no error)=w310) -> (error out=w311:errorcluster)  [unwired: 1 in, 2 out]
        n174 = Release Queue(queue=w304, error in (no error)=w303) -> (error out=w302:errorcluster)  [unwired: 1 in, 2 out]
        n175 = Release Queue(queue=w299, error in (no error)=w300) -> (error out=w301:errorcluster)  [unwired: 1 in, 2 out]
        n176 = Release Queue(queue=w294, error in (no error)=w293) -> (error out=w292:errorcluster)  [unwired: 1 in, 2 out]
        n177 = Release Queue(queue=w289, error in (no error)=w290) -> (error out=w291:errorcluster)  [unwired: 1 in, 2 out]
        n178 = call <vilib>:"Clear Errors.vi"("error in (no error)"=w332) -> ()  [unwired: 6 in, 1 out]
        n179 = call <vilib>:"Clear Errors.vi"("error in (no error)"=w331) -> ()  [unwired: 6 in, 1 out]
        n180 = call <vilib>:"Clear Errors.vi"("error in (no error)"=w322) -> ()  [unwired: 6 in, 1 out]
        n181 = call <vilib>:"Clear Errors.vi"("error in (no error)"=w321) -> ()  [unwired: 6 in, 1 out]
        n182 = call <vilib>:"Clear Errors.vi"("error in (no error)"=w312) -> ()  [unwired: 6 in, 1 out]
        n183 = call <vilib>:"Clear Errors.vi"("error in (no error)"=w311) -> ()  [unwired: 6 in, 1 out]
        n184 = call <vilib>:"Clear Errors.vi"("error in (no error)"=w302) -> ()  [unwired: 6 in, 1 out]
        n185 = call <vilib>:"Clear Errors.vi"("error in (no error)"=w301) -> ()  [unwired: 6 in, 1 out]
        n186 = call <vilib>:"Clear Errors.vi"("error in (no error)"=w292) -> ()  [unwired: 6 in, 1 out]
        n187 = call <vilib>:"Clear Errors.vi"("error in (no error)"=w291) -> ()  [unwired: 6 in, 1 out]
      }
      n188 = control-ref of="Grennich Offset"() -> (w124:refnum<vi>)
      n189 = control-ref of="Use RCVR 1"() -> (w234:refnum<vi>)
      n190 = control-ref of="UPDT COM 1"() -> (w231:refnum<vi>)
      n191 = control-ref of="Use RCVR 2"() -> (w223:refnum<vi>)
      n192 = control-ref of="UPDT COM 2"() -> (w226:refnum<vi>)
      n193 = control-ref of="Use RCVR 3"() -> (w215:refnum<vi>)
      n194 = control-ref of="UPDT COM 3"() -> (w212:refnum<vi>)
      n195 = control-ref of="Use RCVR 4"() -> (w205:refnum<vi>)
      n196 = control-ref of="UPDT COM 4"() -> (w208:refnum<vi>)
      n197 = control-ref of="Use RCVR 5"() -> (w203:refnum<vi>)
      n198 = control-ref of="UPDT COM 5"() -> (w200:refnum<vi>)
      n199 = control-ref of="Use RCVR 6"() -> (w193:refnum<vi>)
      n200 = control-ref of="UPDT COM 6"() -> (w196:refnum<vi>)
      n201 = control-ref of="Use RCVR 7"() -> (w191:refnum<vi>)
      n202 = control-ref of="UPDT COM 7"() -> (w188:refnum<vi>)
      n203 = control-ref of="Use RCVR 8"() -> (w181:refnum<vi>)
      n204 = control-ref of="UPDT COM 8"() -> (w184:refnum<vi>)
      n205 = control-ref of="Use RCVR 9"() -> (w179:refnum<vi>)
      n206 = control-ref of="UPDT COM 9"() -> (w176:refnum<vi>)
      n207 = control-ref of="Use RCVR 10"() -> (w169:refnum<vi>)
      n208 = control-ref of="UPDT COM 10"() -> (w172:refnum<vi>)
      n209 = control-ref of="COM Port 1"() -> (w232:refnum<vi>)
      n210 = control-ref of="COM Port 2"() -> (w225:refnum<vi>)
      n211 = control-ref of="COM Port 3"() -> (w213:refnum<vi>)
      n212 = control-ref of="COM Port 4"() -> (w207:refnum<vi>)
      n213 = control-ref of="COM Port 5"() -> (w201:refnum<vi>)
      n214 = control-ref of="COM Port 6"() -> (w195:refnum<vi>)
      n215 = control-ref of="COM Port 7"() -> (w189:refnum<vi>)
      n216 = control-ref of="COM Port 8"() -> (w183:refnum<vi>)
      n217 = control-ref of="COM Port 9"() -> (w177:refnum<vi>)
      n218 = control-ref of="COM Port 10"() -> (w171:refnum<vi>)
      n219 = control-ref of="A_Off R 2"() -> (w152:refnum<vi>)
      n220 = control-ref of="A_Off R 5"() -> (w149:refnum<vi>)
      n221 = control-ref of="A_Off R 9"() -> (w145:refnum<vi>)
      n222 = control-ref of="Name of RCVR 1"() -> (w233:refnum<vi>)
      n223 = control-ref of="Name of RCVR 2"() -> (w224:refnum<vi>)
      n224 = control-ref of="Last 10 RCVR 2"() -> (w227:refnum<vi>)
      n225 = control-ref of="Name of RCVR 3"() -> (w214:refnum<vi>)
      n226 = control-ref of="A_Off R 3"() -> (w151:refnum<vi>)
      n227 = control-ref of="Name of RCVR 4"() -> (w206:refnum<vi>)
      n228 = control-ref of="A_Off R 4"() -> (w150:refnum<vi>)
      n229 = control-ref of="Name of RCVR 5"() -> (w202:refnum<vi>)
      n230 = control-ref of="Name of RCVR 6"() -> (w194:refnum<vi>)
      n231 = control-ref of="A_Off R 6"() -> (w148:refnum<vi>)
      n232 = control-ref of="Name of RCVR 7"() -> (w190:refnum<vi>)
      n233 = control-ref of="Name of RCVR 8"() -> (w182:refnum<vi>)
      n234 = control-ref of="Name of RCVR 9"() -> (w178:refnum<vi>)
      n235 = control-ref of="Name of RCVR 10"() -> (w170:refnum<vi>)
      n236 = control-ref of="A_Off R 1"() -> (w153:refnum<vi>)
      n237 = control-ref of="A_Off R 8"() -> (w146:refnum<vi>)
      n238 = control-ref of="A_Off R 10"() -> (w144:refnum<vi>)
      n239 = control-ref of="Last 10 RCVR 1"() -> (w229:refnum<vi>)
      n240 = control-ref of="Last 10 RCVR 3"() -> (w211:refnum<vi>)
      n241 = control-ref of="Last 10 RCVR 4"() -> (w209:refnum<vi>)
      n242 = control-ref of="Last 10 RCVR 5"() -> (w199:refnum<vi>)
      n243 = control-ref of="Last 10 RCVR 6"() -> (w197:refnum<vi>)
      n244 = control-ref of="Last 10 RCVR 7"() -> (w187:refnum<vi>)
      n245 = control-ref of="A_Off R 7"() -> (w147:refnum<vi>)
      n246 = control-ref of="Last 10 RCVR 8"() -> (w185:refnum<vi>)
      n247 = control-ref of="Last 10 RCVR 9"() -> (w175:refnum<vi>)
      n248 = control-ref of="Last 10 RCVR 10"() -> (w173:refnum<vi>)
      n249 = Bundle By Name(cluster=w220, "setup save cluster.Base File Path"=w219, "setup save cluster.Time between samples (seconds)"=w218, "setup save cluster.Number of hours To Collect before starting new file"=w217) -> (w216:T3)
      n250 = Build Array(w234, w233, w232, w231, w229, w153, w124) -> (w230:refnum<vi>[])
      n251 = Build Array(w223, w224, w225, w226, w227, w152, w124) -> (w222:refnum<vi>[])
      n252 = Build Array(w215, w214, w213, w212, w211, w151, w124) -> (w210:refnum<vi>[])
      n253 = Build Array(w205, w206, w207, w208, w209, w150, w124) -> (w204:refnum<vi>[])
      n254 = Build Array(w203, w202, w201, w200, w199, w149, w124) -> (w198:refnum<vi>[])
      n255 = Build Array(w193, w194, w195, w196, w197, w148, w124) -> (w192:refnum<vi>[])
      n256 = Build Array(w191, w190, w189, w188, w187, w147, w124) -> (w186:refnum<vi>[])
      n257 = Build Array(w181, w182, w183, w184, w185, w146, w124) -> (w180:refnum<vi>[])
      n258 = Build Array(w179, w178, w177, w176, w175, w145, w124) -> (w174:refnum<vi>[])
      n259 = Build Array(w169, w170, w171, w172, w173, w144, w124) -> (w168:refnum<vi>[])
      n260 = call "single com port capture vi.vi"("unique queue name"="1", "Reference to control Array"=w230) -> ("error out"=w228:errorcluster, "Reference to control Array Out"=w143:refnum<vi>[])  [unwired: 8 in]
      n261 = call "single com port capture vi.vi"("unique queue name"="2", "Reference to control Array"=w222) -> ("error out"=w142:errorcluster, "Reference to control Array Out"=w125:refnum<vi>[])  [unwired: 8 in]
      n262 = call "single com port capture vi.vi"("unique queue name"="3", "Reference to control Array"=w210) -> ("error out"=w141:errorcluster, "Reference to control Array Out"=w126:refnum<vi>[])  [unwired: 8 in]
      n263 = call "single com port capture vi.vi"("unique queue name"="4", "Reference to control Array"=w204) -> ("error out"=w140:errorcluster, "Reference to control Array Out"=w127:refnum<vi>[])  [unwired: 8 in]
      n264 = call "single com port capture vi.vi"("unique queue name"="5", "Reference to control Array"=w198) -> ("error out"=w139:errorcluster, "Reference to control Array Out"=w128:refnum<vi>[])  [unwired: 8 in]
      n265 = call "single com port capture vi.vi"("unique queue name"="6", "Reference to control Array"=w192) -> ("error out"=w138:errorcluster, "Reference to control Array Out"=w129:refnum<vi>[])  [unwired: 8 in]
      n266 = call "single com port capture vi.vi"("unique queue name"="7", "Reference to control Array"=w186) -> ("error out"=w137:errorcluster, "Reference to control Array Out"=w130:refnum<vi>[])  [unwired: 8 in]
      n267 = call "single com port capture vi.vi"("unique queue name"="8", "Reference to control Array"=w180) -> ("error out"=w136:errorcluster, "Reference to control Array Out"=w131:refnum<vi>[])  [unwired: 8 in]
      n268 = call "single com port capture vi.vi"("unique queue name"="9", "Reference to control Array"=w174) -> ("error out"=w135:errorcluster, "Reference to control Array Out"=w132:refnum<vi>[])  [unwired: 8 in]
      n269 = call "single com port capture vi.vi"("unique queue name"="10", "Reference to control Array"=w168) -> ("error out"=w134:errorcluster, "Reference to control Array Out"=w133:refnum<vi>[])  [unwired: 8 in]
      n270 = case shown="Error" w228 {
        frame No Error {
        }
        frame Error {
          n271 = call "Display Message to User14"("Message"="An Error Occurred at RCVR 1 at shutdown.") -> ()  [unwired: 9 in, 2 out]
        }
      }
      n272 = case shown="Error" w142 {
        frame No Error {
        }
        frame Error {
          n273 = call "Display Message to User"("Message"="An Error Occurred at RCVR 2 at shutdown.") -> ()  [unwired: 9 in, 2 out]
        }
      }
      n274 = case shown="Error" w141 {
        frame No Error {
        }
        frame Error {
          n275 = call "Display Message to User2"("Message"="An Error Occurred at RCVR 3 at shutdown.") -> ()  [unwired: 9 in, 2 out]
        }
      }
      n276 = case shown="Error" w140 {
        frame No Error {
        }
        frame Error {
          n277 = call "Display Message to User3"("Message"="An Error Occurred at RCVR 4 at shutdown.") -> ()  [unwired: 9 in, 2 out]
        }
      }
      n278 = case shown="Error" w139 {
        frame No Error {
        }
        frame Error {
          n279 = call "Display Message to User4"("Message"="An Error Occurred at RCVR 5 at shutdown.") -> ()  [unwired: 9 in, 2 out]
        }
      }
      n280 = case shown="Error" w138 {
        frame No Error {
        }
        frame Error {
          n281 = call "Display Message to User5"("Message"="An Error Occurred at RCVR 6 at shutdown.") -> ()  [unwired: 9 in, 2 out]
        }
      }
      n282 = case shown="Error" w137 {
        frame No Error {
        }
        frame Error {
          n283 = call "Display Message to User6"("Message"="An Error Occurred at RCVR 7 at shutdown.") -> ()  [unwired: 9 in, 2 out]
        }
      }
      n284 = case shown="Error" w136 {
        frame No Error {
        }
        frame Error {
          n285 = call "Display Message to User7"("Message"="An Error Occurred at RCVR 8 at shutdown.") -> ()  [unwired: 9 in, 2 out]
        }
      }
      n286 = case shown="Error" w135 {
        frame No Error {
        }
        frame Error {
          n287 = call "Display Message to User8"("Message"="An Error Occurred at RCVR 9 at shutdown.") -> ()  [unwired: 9 in, 2 out]
        }
      }
      n288 = case shown="Error" w134 {
        frame No Error {
        }
        frame Error {
          n289 = call "Display Message to User9"("Message"="An Error Occurred at RCVR 10 at shutdown.") -> ()  [unwired: 9 in, 2 out]
        }
      }
      n290 = for {
        tunnel: w143 -> [w253] mode=indexing
        n291 = Close Reference(reference=w253) -> ()  [unwired: 1 in, 1 out]
      }
      n292 = for {
        tunnel: w125 -> [w251] mode=indexing
        n293 = Close Reference(reference=w251) -> ()  [unwired: 1 in, 1 out]
      }
      n294 = for {
        tunnel: w126 -> [w249] mode=indexing
        n295 = Close Reference(reference=w249) -> ()  [unwired: 1 in, 1 out]
      }
      n296 = for {
        tunnel: w127 -> [w247] mode=indexing
        n297 = Close Reference(reference=w247) -> ()  [unwired: 1 in, 1 out]
      }
      n298 = for {
        tunnel: w128 -> [w245] mode=indexing
        n299 = Close Reference(reference=w245) -> ()  [unwired: 1 in, 1 out]
      }
      n300 = for {
        tunnel: w129 -> [w243] mode=indexing
        n301 = Close Reference(reference=w243) -> ()  [unwired: 1 in, 1 out]
      }
      n302 = for {
        tunnel: w130 -> [w241] mode=indexing
        n303 = Close Reference(reference=w241) -> ()  [unwired: 1 in, 1 out]
      }
      n304 = for {
        tunnel: w131 -> [w239] mode=indexing
        n305 = Close Reference(reference=w239) -> ()  [unwired: 1 in, 1 out]
      }
      n306 = for {
        tunnel: w132 -> [w237] mode=indexing
        n307 = Close Reference(reference=w237) -> ()  [unwired: 1 in, 1 out]
      }
      n308 = for {
        tunnel: w133 -> [w235] mode=indexing
        n309 = Close Reference(reference=w235) -> ()  [unwired: 1 in, 1 out]
      }
    }
    frame #2 {
      w495 = T6 3 items=["User Home"=0, "User Desktop"=1, "User Documents"=2, "User Application Data"=3, "User Preferences"=4, "User Temporary"=5, "Public Documents"=6, "Public Application Data"=7, "Public Preferences"=8, "Public Cache"=13, "System Core Libraries"=9, "System Installed Libraries"=10, "Application Files"=11, "Boot Volume Root"=12] ("system directory type")
      # "Close out steps"
      n310 = call <vilib>:"Get System Directory.vi"("system directory type"=w495) -> ("system directory"=w492:path)  [unwired: 10 in]
      n311 = Build Path(base path=w492, name or relative path="Com2TXT.confg") -> (appended path=w497:path)
      n312 = Write to Binary File(file (use dialog)=w497, data=w487, 9:T4."little-endian" ("byte order (0:big-endian, network order)")) -> (refnum out=w494:refnum<file>, error out=w493:errorcluster)  [unwired: 3 in, 1 out]
      n313 = Close File(refnum=w494, error in=w493) -> (error out=w499:errorcluster)  [unwired: 1 out]
      n314 = call <vilib>:"Simple Error Handler.vi"("error in (no error)"=w499) -> ("error out"=w490:errorcluster)  [unwired: 4 in, 4 out]
      n315 = call <vilib>:"Clear Errors.vi"("error in (no error)"=w490) -> ("error out"=w498:errorcluster)  [unwired: 6 in]
      n316 = property class="App"(error in=w498) -> (error out=w488:errorcluster, "App.Kind"=w489:T18)  [unwired: 1 in, 1 out]
      n317 = case shown="\"Development System\"" w489 {
        tunnel: w488 -> [_ _ _ _ _ _ _]
        frame "invalid app kind", Default {
        }
        frame "Development System" {
        }
        frame "Run Time System" {
          n318 = Quit LabVIEW() -> ()  [unwired: 1 in]
        }
        frame "Student Edition" {
        }
        frame "Embedded LabVIEW" {
        }
        frame "Evaluation" {
        }
        frame "Custom" {
        }
      }
    }
  }
